vi "getAttribute_Number_Complex128.vi"(7 "object":string, 8 "error in (no error)":errorcluster, 10 "attribute":string, 11 "LabVIEW-Python-Interface in":refnum<class "PyLVi.lvclass">) -> (0 "error out":errorcluster, 2 "data":cdb, 3 "LabVIEW-Python-Interface out":refnum<class "PyLVi.lvclass">)   [LabVIEW 2016, in "PyLVi.lvlib" / "PyLVi.lvclass"]
uses:
  PyLVi.lvclass
  return_get/getReturn_Number_Complex128.vi
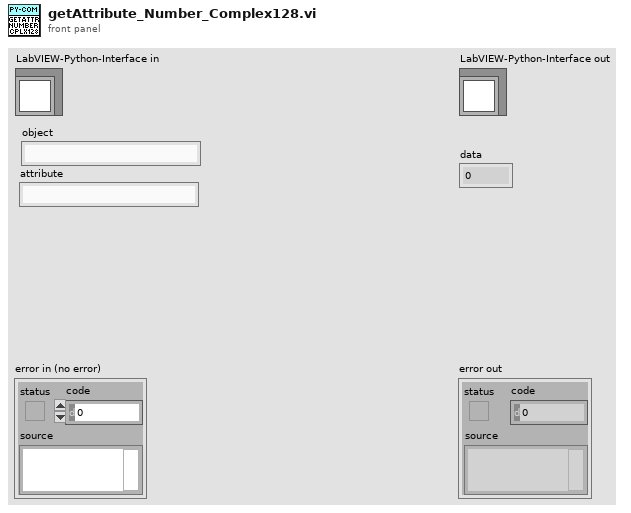
[diagram p1: front panel]
types:
  T1 = typedef "PyLVi.lvlib/PyLVi.lvclass/ArgumentStructure.ctl" = cluster{"descriptor structure":T2, "data string":string}
  T2 = typedef "PyLVi.lvlib/PyLVi.lvclass/DescriptorStructure.ctl" = cluster{"argtype":string, "dtype":string, "shape":u32[], "argname":string}
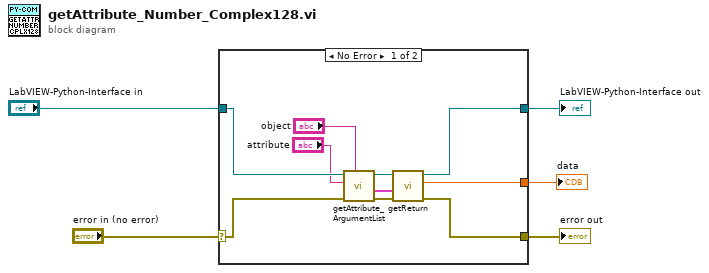
[diagram p0: block diagram]
diagram:
  n1 = case shown="No Error" "error in (no error)" {
    selector: "error in (no error)" -> [w12 w17]
    tunnel: [w7 w17] -> w4
    tunnel: [w8 w16] -> w2
    tunnel: "LabVIEW-Python-Interface in" -> [w15 w16]
    tunnel: [w6 _] -> w1
    frame No Error {
      n2 = call "getAttribute_ArgumentList.vi"("object"="object", "error in (no error)"=w12, "attribute"="attribute", "LabVIEW-Python-Interface in"=w15) -> ("error out"=w9:errorcluster, "return list"=w10:T1[], "LabVIEW-Python-Interface out"=w11:refnum<class "PyLVi.lvclass">)  [unwired: 5 in]
      n3 = call-poly "getReturn.vi"("error in (no error)"=w9, "return list in"=w10, "LabVIEW-Python-Interface in"=w11) -> ("error out"=w7:errorcluster, "data out"=w6:cdb, "LabVIEW-Python-Interface out"=w8:refnum<class "PyLVi.lvclass">)  [unwired: 5 in, 1 out]
    }
    frame Error {
    }
  }
  "error out" <- w4
  "LabVIEW-Python-Interface out" <- w2
  "data" <- w1
